vi "Preset FAIL CONTINUITY.vi"(8 "error in (no error)":errorcluster, 11 "VISA resource in":refnum<visa-resource-name>) -> (0 "error out":errorcluster, 3 "VISA resource out":refnum<visa-resource-name>)   [LabVIEW 2025, in "Chroma 19572.lvlib"]
doc: "This VI writes to the instrument the AC-V FREQ. value."
uses:
  <instrlib>/Chroma 19572/Chroma 19572.lvlib
panel:
  in  "on/off":u16(ring) items=["OFF", "ON"]
  # "Set Fail Continuity state\nON: test continues\nOFF: stop test"
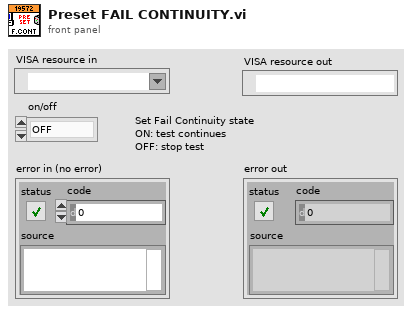
[diagram p1: front panel]
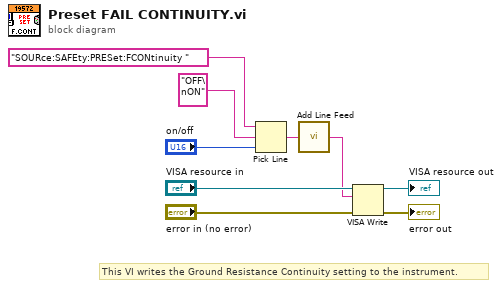
[diagram p0: block diagram]
diagram:
  # "This VI writes the Ground Resistance Continuity setting to the instrument."
  n1 = Pick Line(string ("")="SOURce:SAFEty:PRESet:FCONtinuity ", multi-line string="OFF\nON" ("format string"), line index="on/off") -> (output string=w4:string)
  n2 = call <instrlib>:"Add Line Feed.vi"("Command string"=w4) -> ("Concatenated string"=w7:string)  [unwired: 4 in]
  n3 = VISA Write(VISA resource name="VISA resource in", write buffer=w7, error in (no error)="error in (no error)") -> (VISA resource name out=→"VISA resource out":refnum<visa-resource-name>, error out=→"error out":errorcluster)  [unwired: 1 out]
